vi "Main.vi"(11 "Module Admin":refnum<class "Delacor_lib_QMH_Module Admin.lvclass">) -> ()   [LabVIEW 2020, in "Rename As Application UI.lvlib"]
doc: "This template is based off of the Queued Message Handler design pattern and the Queued Message Handler project template that ships with LabVIEW.\n\nThe main difference is that the queue is private to this module and communication between modules is performed via Broadcast and Request events.\n\nRequest events are wrapped in public API methods and are handled in the Event Handling Loop (EHL) of this VI. Any module can register for Broadcast events sent by this module. The EHL generates messages based on user interface actions.\n\nThe Message Handling Loop (MHL) processes messages generated by the EHL, or by other messages. The messages are string values, so new messages can be added easily to the Message Cases case structure in the MHL. Each message cluster can also provide an optional value for Message Data, which is a variant that can be converted to whatever message-specific data is required.\n_____\nBased on DQMH Project Template 6.1.0.94.\n\n<b>Note:</b> This VI was modified by the <b>Validate DQMH Module</b> tool to add a call to the Error Reported VI at the end of the 'Exit' MHL frame."
uses:
  Rename As Application UI.lvlib
  <vilib>/Delacor/Delacor QMH/Libraries/Module Admin_class/Delacor_lib_QMH_Module Admin.lvclass
  Module Data--cluster.ctl
  Configuration/Configuration--cluster.ctl
  <vilib>/Delacor/Delacor QMH/Libraries/Message Queue_class/Delacor_lib_QMH_Message Queue.lvclass/Delacor_lib_QMH_Message Queue.ctl
  Stop Argument--cluster.ctl
  <vilib>/Utility/miscctls.llb/LVPointTypeDef.ctl
  <vilib>/Delacor/Delacor QMH/Libraries/Module Admin_class/Delacor_lib_QMH_Module Admin.lvclass/Delacor_lib_QMH_Module Admin.ctl
  Configuration/Configuration.lvclass
  Configuration/Configuration.lvclass/Configuration.ctl
  <vilib>/Delacor/Delacor QMH/Libraries/Message Queue_class/Delacor_lib_QMH_Enqueue Message (Single).vi
  <vilib>/Delacor/Delacor QMH/Libraries/Module Admin_class/Delacor_lib_QMH_Get External Launch.vi
  Configuration/Get Configuration.vi
  <vilib>/Utility/error.llb/Error Cluster From Error Code.vi
  <vilib>/ErrorRing/Error Ring.xnode
  <vilib>/Delacor/Delacor QMH/Libraries/Message Queue_class/Delacor_lib_QMH_Message Queue.lvclass
  <vilib>/Peloton/Pelobuttons/Pelobuttons_lib_Pelobuttons.lvlib
  <vilib>/Peloton/Peloton Config/DCFG Framework/Peloton_lib_DCFG Framework.lvlib
  Rename As Application Shared/Rename as Application Shared.lvlib
  <vilib>/Peloton/Peloton Config/DCFG Framework/Configuration_class/Configuration.lvclass
panel:
  out "version":string
  in  "About":bool
  in  "Configuration":bool
  in  "Random Path":path
  out "error out":errorcluster
  in  "Simulate MHL Error":bool
  in  "Simulate EHL Error":bool
  # "This will be the main UI for your application.\nIf you are running as an executable and you want to run in debug mode, drag the exe to the cmd prompt and\nadd the argument -- debug.\nThe project already has a build specification."
  # "When editing this GUI, use Pelobuttons."
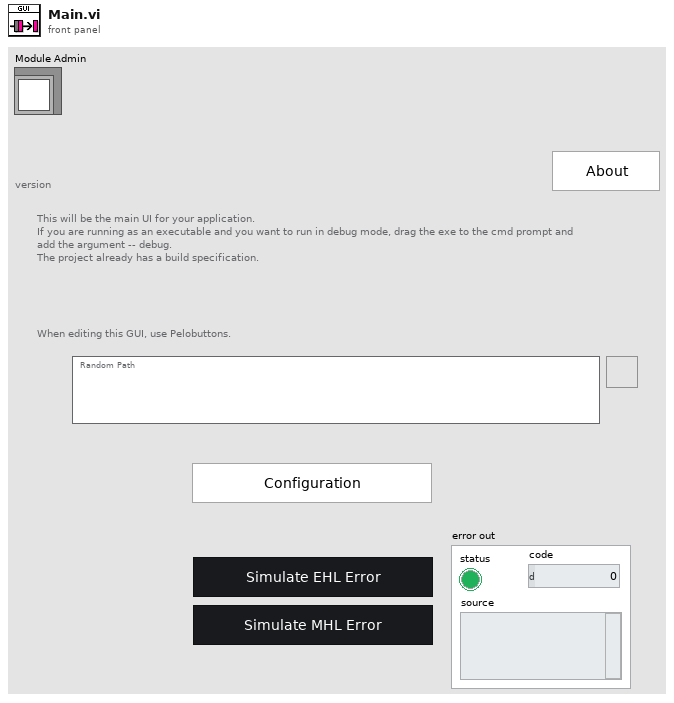
[diagram p1: front panel]
types:
  T1 = typedef "Rename As Application UI.lvlib/Request Events--cluster.ctl" = cluster{"Stop Module":refnum<user-event>, "Show Panel":refnum<user-event>, "Hide Panel":refnum<user-event>, "Get Module Execution Status":refnum<user-event>, "Show Diagram":refnum<user-event>}
  T2 = typedef "Peloton_lib_DCFG Framework.lvlib/Broadcast Events--cluster.ctl" = cluster{"Module Did Init":refnum<user-event>, "Status Updated":refnum<user-event>, "Error Reported":refnum<user-event>, "Module Did Stop":refnum<user-event>, "Update Module Execution Status":refnum<user-event>, "View Changed":refnum<user-event>, "Main Window Closed":refnum<user-event>, "Configuration Committed":refnum<user-event>, "Configuration Canceled":refnum<user-event>, "Views List Updated":refnum<user-event>, "Config Folder Path Updated":refnum<user-event>}
  T3 = typedef "Rename As Application UI.lvlib/Module Data--cluster.ctl" = cluster{"Status":string, "Configuration":T4}
  T4 = typedef "Rename As Application UI.lvlib/Configuration.lvclass/Configuration--cluster.ctl" = cluster{"Random Path":path}
  T5 = enum32{"invalid lock state", "Not Locked", "Locked (No Password)", "Password-protected"}
  T6 = typedef "Rename As Application UI.lvlib/Stop Argument--cluster.ctl" = cluster{"Origin":string, "Exit via Stop Module Req?":bool, "Wait for Module to stop?":bool}
  T7 = typedef "LVPointTypeDef.ctl" = cluster{"Horizontal":i16, "Vertical":i16}
  T8 = enum32{"Invalid", "Standard", "Closed", "Hidden", "Minimized", "Maximized"}
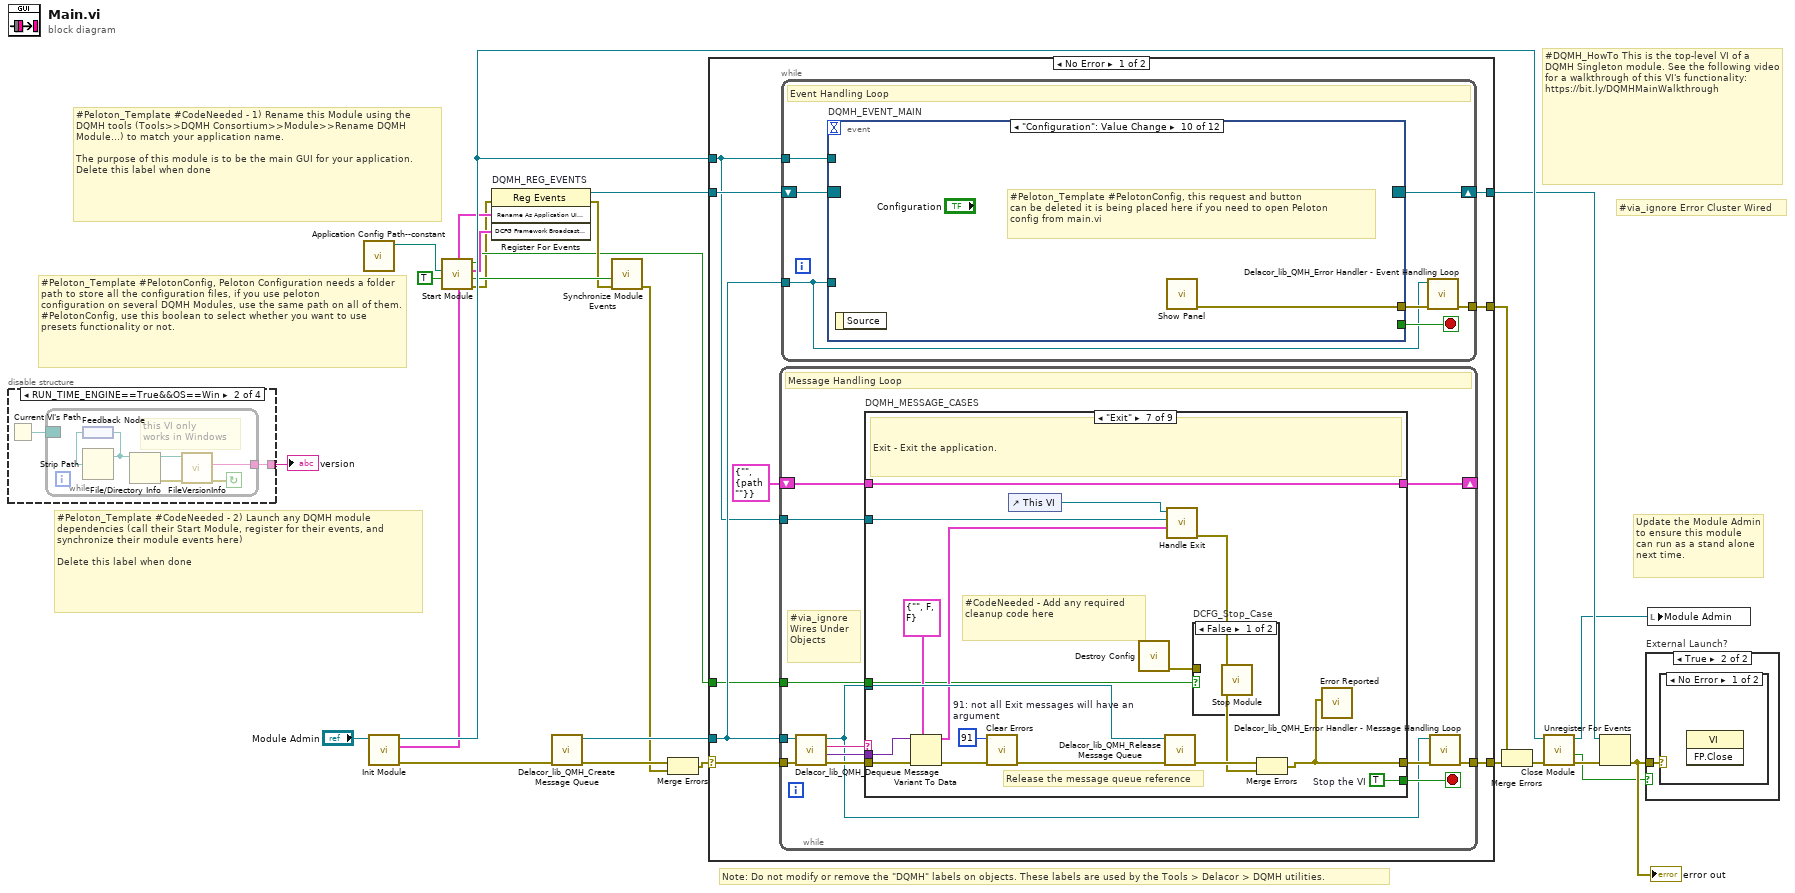
[diagram p0: block diagram]
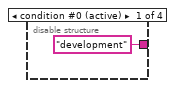
[diagram p2: hidden frame]
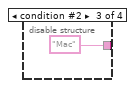
[diagram p3: hidden frame]
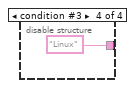
[diagram p4: hidden frame]
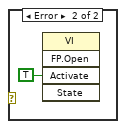
[diagram p6: hidden frame]
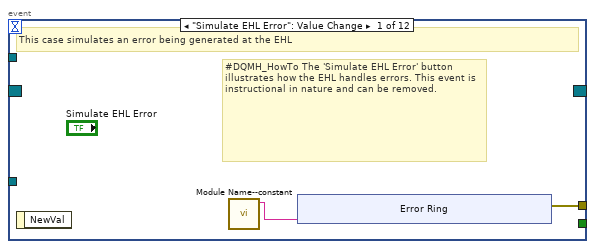
[diagram p7: hidden frame]
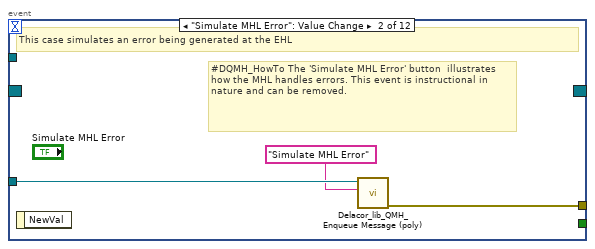
[diagram p8: hidden frame]
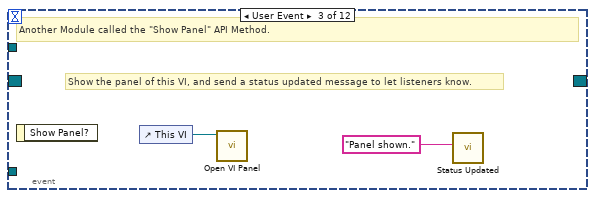
[diagram p9: hidden frame]
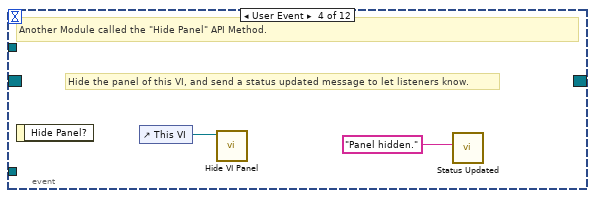
[diagram p10: hidden frame]
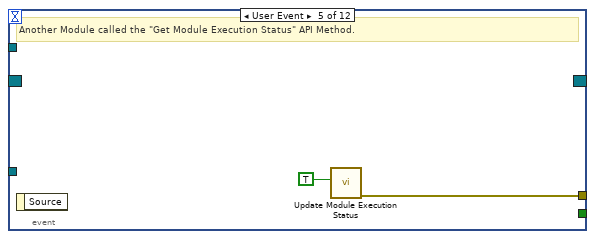
[diagram p11: hidden frame]
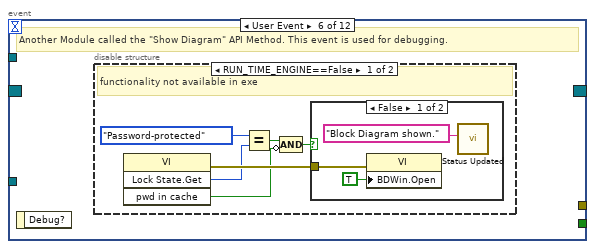
[diagram p12: hidden frame]
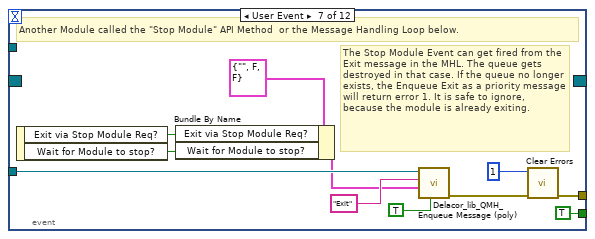
[diagram p15: hidden frame]
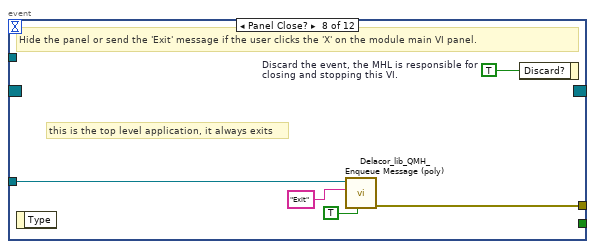
[diagram p16: hidden frame]
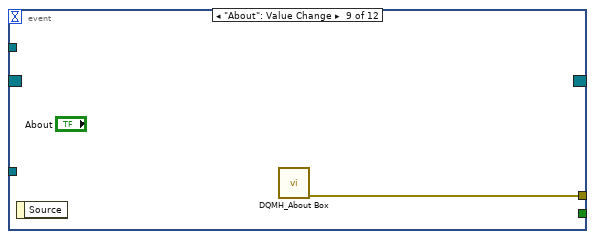
[diagram p17: hidden frame]
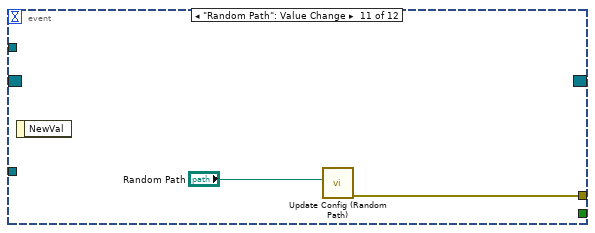
[diagram p18: hidden frame]
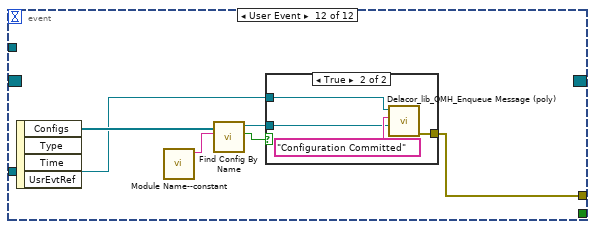
[diagram p19: hidden frame]
diagram:
  # "#Peloton_Template #PelotonConfig, Peloton Configuration needs a folder path to store all the configuration files, if you use peloton\nconfiguration on several DQMH Modules, use the same path on all of them.\n#PelotonConfig, use this boolean to select whether you want to use\npresets functionality or not."
  # "#via_ignore Error Cluster Wired"
  # "#Peloton_Template #CodeNeeded - 2) Launch any DQMH module dependencies (call their Start Module, register for their events, and synchronize their module events here)\n\nDelete this label when done"
  # "#Peloton_Template #CodeNeeded - 1) Rename this Module using the DQMH tools (Tools>>DQMH Consortium>>Module>>Rename DQMH Module...) to match your application name.\n\nThe purpose of this module is to be the main GUI for your application.\nDelete this label when done"
  # "#DQMH_HowTo This is the top-level VI of a DQMH Singleton module. See the following video for a walkthrough of this VI's functionality: https://bit.ly/DQMHMainWalkthrough"
  # "Note: Do not modify or remove the \"DQMH\" labels on objects. These labels are used by the Tools > Delacor > DQMH utilities."
  # "Update the Module Admin to ensure this module can run as a stand alone next time."
  n1 = disable-structure "Conditional Disable Structure" shown="RUN_TIME_ENGINE==True&&OS==Win" {
    disable-tunnel: ["development" w27 "Mac" "Linux"] -> w9
    frame condition #0 (active) {
    }
    frame condition #1 {
      n2 = Current VI's Path() -> (path=w28:path)
      n3 = while {
        border: w28 -> [_]
        tunnel: [w29] -> w27
        stop <- w33 continue-if-true
        # "this VI only \nworks in Windows"
        n4 = feedback #1() -> (w32:path)
        n5 = Strip Path(path=w32) -> (stripped path=w31:path)  [unwired: 1 out]
        n6 = feedback-in #1(w31) -> ()
        n7 = File/Directory Info(path=w31) -> (path out=w30:path, error out=w34:errorcluster)  [unwired: 1 in, 5 out]
        n8 = call <vilib>:"FileVersionInfo.vi"("error in (no error)"=w34, "Application Path in"=w30) -> ("error out"=w33:errorcluster, "File Version Info"=w29:string)  [unwired: 6 in, 2 out]
      }
    }
    frame condition #2 {
    }
    frame condition #3 {
    }
  }
  "version" <- w9
  n9 = call "Application Config Path--constant.vi"() -> ("File Path"=w2:path)  [unwired: 11 in]
  n10 = call "Init Module.vi"("Singleton Module Admin in"="Module Admin") -> ("error out"=w24:errorcluster, "Rename As Application UI Request Events"=w14:T1, "Singleton Module Admin out"=w17:refnum<class "Delacor_lib_QMH_Module Admin.lvclass">)  [unwired: 8 in]
  n11 = call <vilib>:"Start Module.vi"("Enable Presets (F)"=TRUE, "Config Folder"=w2) -> ("error out"=w1:errorcluster, "Wait for Event Sync?"=w7:bool, "DCFG Framework Broadcast Events"=w8:T2, "Module Was Already Running?"=w4:bool)  [unwired: 6 in]
  n12 = register-events "DQMH_REG_EVENTS"(error in=w1, w14, w8) -> (reference out=w15:refnum<event-registration>, error out=w6:errorcluster)  [unwired: 1 in]
  n13 = call <vilib>:"Delacor_lib_QMH_Create Message Queue.vi"("error in"=w24) -> ("error out"=w19:errorcluster, "Message Queue"=w13:refnum<class "Delacor_lib_QMH_Message Queue.lvclass">)  [unwired: 9 in]
  n14 = call <vilib>:"Synchronize Module Events.vi"("error in (no error)"=w6, "Wait for Event Sync?"=w7) -> ("error out"=w5:errorcluster)  [unwired: 9 in]
  n15 = Merge Errors(w19, w5) -> (w18:errorcluster)
  n16 = case shown="No Error" w18 {
    selector: w18 -> [w43 w229]
    tunnel: [w45 w228] -> w25
    tunnel: [w42 w227] -> w16
    tunnel: w15 -> [w40 w227]
    tunnel: w13 -> [w39 w222]
    tunnel: [w44 _] -> w22
    tunnel: w17 -> [w38 w223]
    tunnel: w4 -> [w37 w221]
    frame No Error {
      n17 = while {
        tunnel: w39 -> [w113]
        shift-right: [w117] -> _
        shift-left: T3 {"Status"="", "Configuration"={"Random Path"=path ""}} ("Data Cluster") -> [w118]
        tunnel: w43 -> [w121]
        tunnel: [w119] -> w45
        tunnel: w38 -> [w111]
        tunnel: w37 -> [w110]
        stop <- w116 stop-if-true
        # "#via_ignore Wires Under Objects"
        # "Message Handling Loop"
        n18 = call-dynamic "Delacor_lib_QMH_Dequeue Message.vi"("error in"=w121, "Message Queue in"=w113) -> ("error out"=w120:errorcluster, "Message Data"=w114:variant, "Message"=w115:string, "Message Queue out"=w112:refnum<class "Delacor_lib_QMH_Message Queue.lvclass">)  [unwired: 6 in]
        n19 = case "DQMH_MESSAGE_CASES" shown="\"Exit\"" w115 {
          selector: w115 -> [_ _ _ _ _ _ _ w199 _]
          tunnel: w112 -> [_ _ _ _ _ w167 w190 _ _]
          tunnel: w120 -> [w143 w147 w150 w152 w157 w174 w197 w201 w220]
          tunnel: [w142 w147 w149 w152 w156 w170 w194 w202 w217] -> w122
          tunnel: w118 -> [w129 w146 w148 w151 w154 w169 w189 w200 w219]
          tunnel: [w128 w146 w148 w151 w154 w169 w189 w200 w218] -> w117
          tunnel: [_ _ _ _ _ _ w188 _ _] -> w116
          tunnel: w114 -> [_ _ _ _ _ w168 w191 _ w216]
          tunnel: w111 -> [w134 _ _ _ _ w166 w184 _ _]
          tunnel: w110 -> [_ _ _ _ _ _ w181 _ _]
          frame "Initialize" {
            # "#CodeNeeded - Initialize the appearance of the front panel."
            # "Initialize - Any operation that needs to be done before the module can receive messages. Synchronize Caller Events.vi will inform Start Module.vi that the module has launched and is ready to receive messages. Module Did Init.vi will broadcast that the module initialized."
            n20 = call "Synchronize Caller Events.vi"("error in (no error)"=w143, "Singleton Module Admin in"=w134) -> ("error out"=w125:errorcluster, "Singleton Module Admin out"=w131:refnum<class "Delacor_lib_QMH_Module Admin.lvclass">)  [unwired: 8 in]
            n21 = property on="Property Node" class="Module Admin"(reference=w131) -> ("Accessors:External Launch"=w138:bool)  [unwired: 1 in, 2 out]
            n22 = flat-sequence {
              tunnel: w125 -> [_]
              frame #0 {
                n23 = call <vilib>:"Brand UI - FP.vi"() -> ()  [unwired: 12 in]
              }
            }
            n24 = call "Init Config.vi"("error in"=w125) -> ("error out"=w126:errorcluster, "Configuration"=w124:T4)  [unwired: 9 in]
            n25 = Select(t=T8."Hidden" ("State"), s=w138, f=T8."Standard" ("State")) -> (s? t:f=w135:T8)
            n26 = call "Module Name--constant.vi"() -> ("Module Name"=w141:string)  [unwired: 11 in]
            n27 = Unbundle By Name(w124) -> ("Random Path"=w123:path)
            n28 = property on="Property Node" class="VI"("Front Panel.Title"=w141) -> (reference out=w140:refnum<vi>, error out=w145:errorcluster)  [unwired: 2 in]
            n29 = call "Module Name--constant.vi"() -> ("Module Name"=w132:string)  [unwired: 11 in]
            n30 = invoke on="Invoke Node" class="VI" method="FP.Open"(reference=w140, error in=w145, "State"=w135) -> (reference out=w139:refnum<vi>, error out=w144:errorcluster)  [unwired: 2 in, 3 out]
            n31 = Bundle By Name(cluster=w129, "Status"="Init", "Configuration"=w124) -> (w128:T3)
            n32 = local write "Random Path"(w123) -> ()
            n33 = call "Module Did Init.vi"("error in (no error)"=w126, "Initialized?"=TRUE, "Origin"=w132) -> ("error out"=w142:errorcluster)  [unwired: 8 in]
            n34 = invoke on="Invoke Node" class="VI" method="FP.Center"(reference=w139, error in=w144) -> ()  [unwired: 1 in, 3 out]
            n35 = property on="Pane" class="Pane"("Origin"=T7 {"Horizontal"=0, "Vertical"=0}) -> ()  [unwired: 2 in, 2 out]
          }
          frame "---Module Specific---" {
            # "Separator -- The following cases handle messages specific to this Module."
          }
          frame "---Copy This Frame---" {
            # "Duplicate this frame when creating new messages.  Change this comment in the duplicated frame to describe this message."
            n36 = Merge Errors(w150) -> (w149:errorcluster)
          }
          frame "---Exit and Error Handling---" {
            # "Separator - The following cases handle errors and exit messages."
          }
          frame "Simulate MHL Error" {
            # "#DQMH_HowTo The 'Simulate MHL Error' button  illustrates how the MHL handles errors. This event is instructional in nature and can be removed."
            # "Simulate an error occurring at the MHL"
            n37 = call "Module Name--constant.vi"() -> ("Module Name"=w153:string)  [unwired: 11 in]
            n38 = xnode ("Error Ring")("parameter 0"=w153) -> ("error out"=w155:errorcluster)
            n39 = Merge Errors(w157, w155) -> (w156:errorcluster)
          }
          frame "Error" {
            # "#CodeRecommended - If you ever change the name of this \"Error\" message, you'll need to update the name in the Check Loop Error.vi as well."
            # "#CodeRecommended - If the module is running in standalone mode (External Launch = FALSE), this code will pop up an error dialog and call the 'Exit' message if an error occurs. Add more fine-grained error handling here."
            # "Error - Check the error message data and respond accordingly. This message is sent by the \"Error Handler\" VIs at the end of each loop in this application."
            n40 = property on="Property Node" class="Module Admin"(reference=w166) -> ("Accessors:External Launch"=w165:bool)  [unwired: 1 in, 2 out]
            n41 = Variant To Data(error in=w174, type=errorcluster {"status"=FALSE, "code"=0, "source"=""} ("error constant"), Variant=w168) -> (data=w175:errorcluster, error out=w172:errorcluster)
            n42 = call "Error Reported.vi"("Error"=w175) -> ()  [unwired: 10 in, 1 out]
            n43 = case shown="False" w165 {
              tunnel: [w180 _] -> w171
              tunnel: w167 -> [w178 _]
              tunnel: w175 -> [w179 _]
              frame False {
                # "If the module is running standalone, then pop up an error dialog and call the \"Exit\" message."
                n44 = call <vilib>:"Simple Error Handler.vi"("error in (no error)"=w179) -> ()  [unwired: 4 in, 5 out]
                n45 = call-poly <vilib>:"Delacor_lib_QMH_Enqueue Message (poly).vi"("Priority Message? (F)"=TRUE, "Message"="Exit", "Message Queue in"=w178) -> ("error out"=w180:errorcluster)  [unwired: 7 in, 1 out]
              }
              frame True {
                # "If the module was launched externally, calling the Error Reported broadcast VI is the only action performed by the \"Error\" message. The module's caller can then process the error appropriately."
              }
            }
            n46 = Merge Errors(w172, w171) -> (w170:errorcluster)
            n47 = local write "error out"(w170) -> ()
          }
          frame "Exit" {
            w187 = 91  # 91: not all Exit messages will have an argument
            w188 = TRUE  # Stop the VI
            # "Release the message queue reference"
            # "#CodeNeeded - Add any required cleanup code here"
            # "Exit - Exit the application."
            n48 = Variant To Data(error in=w197, type=T6 {"Origin"="", "Exit via Stop Module Req?"=FALSE, "Wait for Module to stop?"=FALSE} ("Stop Argument"), Variant=w191) -> (data=w185:T6, error out=w193:errorcluster)
            n49 = call <vilib>:"Clear Errors.vi"("error in (no error)"=w193, "specific error code to clear (0: all)"=w187) -> ("error out"=w196:errorcluster)  [unwired: 4 in, 1 out]
            n50 = control-ref of="This VI"() -> (w183:refnum<vi>)
            n51 = call "Destroy Config.vi"() -> ("error out"=w182:errorcluster)  [unwired: 11 in]
            n52 = call-dynamic "Delacor_lib_QMH_Release Message Queue.vi"("error in"=w196, "Message Queue"=w190) -> ("error out"=w195:errorcluster)  [unwired: 9 in]
            n53 = call "Handle Exit.vi"("Stop Argument"=w185, "Admin in"=w184, "VI reference"=w183) -> ("error out"=w192:errorcluster)  [unwired: 7 in, 1 out]
            n54 = case "DCFG_Stop_Case" shown="False" w181 {
              tunnel: w182 -> [_ _]
              frame False {
                n55 = call <vilib>:"Stop Module.vi"() -> ()  [unwired: 11 in, 1 out]
              }
              frame True {
                # "Let DCFG Running if it was already running"
              }
            }
            n56 = Merge Errors(w195, w192) -> (w194:errorcluster)
            n57 = call "Error Reported.vi"("Error"=w194) -> ()  [unwired: 10 in, 1 out]
          }
          frame Default {
            # "'Default' case only runs if there is a message that isn't defined in any of the other cases.  Output a programming error."
            n58 = call "Module Name--constant.vi"() -> ("Module Name"=w198:string)  [unwired: 11 in]
            n59 = xnode ("Error Ring")("parameter 0"=w199, "parameter 1"=w198) -> ("error out"=w203:errorcluster)
            n60 = Merge Errors(w201, w203) -> (w202:errorcluster)
          }
          frame "Configuration Committed" {
            w215 = refnum<class "Configuration.lvclass"> refnum  # Module_Config_Class
            n61 = Variant To Data(error in=w220, type=w215, Variant=w216) -> (data=w214:refnum<class "Configuration.lvclass">, error out=w217:errorcluster)
            n62 = property on="Property Node" class="Config"(reference=w214) -> ("Accessors:Configuration"=w212:T4)  [unwired: 1 in, 2 out]
            n63 = Bundle By Name(cluster=w219, "Configuration"=w212) -> (w218:T3)
            n64 = Unbundle By Name(w212) -> ("Random Path"=w213:path)
            n65 = local write "Random Path"(w213) -> ()
          }
        }
        n66 = call-dynamic "Delacor_lib_QMH_Error Handler - Message Handling Loop.vi"("error in"=w122, "Message Queue in"=w112) -> ("dup error in"=w119:errorcluster)  [unwired: 8 in, 1 out]
      }
      n67 = while {
        tunnel: w39 -> [w46]
        shift-right: [w49] -> w42
        shift-left: w40 -> [w50]
        tunnel: [w51] -> w44
        tunnel: w38 -> [w47]
        stop <- w48 stop-if-true
        # "Event Handling Loop"
        n68 = event "DQMH_EVENT_MAIN" shown="[9] \"Configuration\": Value Change" {
          selector: w50 -> [_ _ _ _ _ _ _ _ _ _ _ _]
          dyn-events: [_ _ _ _ _ _ _ _ _ _ _ _] -> w49
          timeout: _ -> [_ _ _ _ _ _ _ _ _ _ _ _]
          tunnel: [_ _ _ _ _ _ TRUE ("Discard?") _ _ _ _ _] -> w48
          tunnel: w46 -> [_ w63 _ _ _ _ w86 w93 _ _ _ w103]
          tunnel: [w54 w64 _ _ w70 _ w89 w95 w96 w97 w98 w105] -> w52
          tunnel: w47 -> [_ _ _ _ _ _ _ _ _ _ _ _]
          event "Simulate EHL Error": Value Change {
            # "#DQMH_HowTo The 'Simulate EHL Error' button  illustrates how the EHL handles errors. This event is instructional in nature and can be removed."
            # "This case simulates an error being generated at the EHL"
            n69 = event-data() -> ()  [unwired: 1 in, 1 out]
            n70 = call "Module Name--constant.vi"() -> ("Module Name"=w53:string)  [unwired: 11 in]
            n71 = xnode ("Error Ring")("parameter 0"=w53) -> ("error out"=w54:errorcluster)
          }
          event "Simulate MHL Error": Value Change {
            # "#DQMH_HowTo The 'Simulate MHL Error' button  illustrates how the MHL handles errors. This event is instructional in nature and can be removed."
            # "This case simulates an error being generated at the EHL"
            n72 = event-data() -> ()  [unwired: 1 in, 1 out]
            n73 = call-poly <vilib>:"Delacor_lib_QMH_Enqueue Message (poly).vi"("Message"="Simulate MHL Error", "Message Queue in"=w63) -> ("error out"=w64:errorcluster)  [unwired: 8 in, 1 out]
          }
          event User Event {
            # "Show the panel of this VI, and send a status updated message to let listeners know."
            # "Another Module called the \"Show Panel\" API Method."
            n74 = event-data() -> ()  [unwired: 1 in, 1 out]
            n75 = control-ref of="This VI"() -> (w66:refnum<vi>)
            n76 = call "Open VI Panel.vi"("VI"=w66) -> ()  [unwired: 10 in, 1 out]
            n77 = call "Status Updated.vi"("Status"="Panel shown." ("format string")) -> ()  [unwired: 10 in, 1 out]
          }
          event User Event {
            # "Hide the panel of this VI, and send a status updated message to let listeners know."
            # "Another Module called the \"Hide Panel\" API Method."
            n78 = event-data() -> ()  [unwired: 1 in, 1 out]
            n79 = control-ref of="This VI"() -> (w68:refnum<vi>)
            n80 = call "Hide VI Panel.vi"("VI"=w68) -> ()  [unwired: 10 in, 1 out]
            n81 = call "Status Updated.vi"("Status"="Panel hidden." ("format string")) -> ()  [unwired: 10 in, 1 out]
          }
          event User Event {
            # "Another Module called the \"Get Module Execution Status\" API Method."
            n82 = event-data() -> ()  [unwired: 1 in, 1 out]
            n83 = call "Update Module Execution Status.vi"("Running?"=TRUE) -> ("error out"=w70:errorcluster)  [unwired: 10 in]
          }
          event User Event {
            # "Another Module called the \"Show Diagram\" API Method. This event is used for debugging."
            n84 = event-data() -> ()  [unwired: 1 in, 1 out]
            n85 = disable-structure shown="RUN_TIME_ENGINE==False" {
              frame condition #0 (active) {
                # "functionality not available in exe"
                n86 = invoke on="Invoke Node" class="VI" method="Lock State.Get"() -> (error out=w76:errorcluster, "Get Lock State"=w75:T5, "pwd in cache"=w72:bool)  [unwired: 4 in, 1 out]
                n87 = Equal?(x=T5."Password-protected", y=w75) -> (x = y?=w73:bool)
                n88 = Compound Arithmetic op=AND(w73, invert w72) -> (w71:bool)
                n89 = case shown="False" w71 {
                  tunnel: w76 -> [w79 _]
                  frame False {
                    n90 = property on="Property Node" class="VI"(error in=w79, "BDWin.Open"=TRUE ("Block Diagram Window:Open")) -> ()  [unwired: 1 in, 2 out]
                    n91 = call "Status Updated.vi"("Status"="Block Diagram shown." ("format string")) -> ()  [unwired: 10 in, 1 out]
                  }
                  frame True {
                    # "Password-protected VI, and the password is not in the cache. Do not show the diagram."
                  }
                }
              }
              frame condition #1 {
              }
            }
          }
          event User Event {
            # "The Stop Module Event can get fired from the Exit message in the MHL. The queue gets destroyed in that case. If the queue no longer exists, the Enqueue Exit as a priority message will return error 1. It is safe to ignore, because the module is already exiting."
            # "Another Module called the \"Stop Module\" API Method  or the Message Handling Loop below."
            n92 = event-data() -> ("Exit via Stop Module Req?"=w82:bool, "Wait for Module to stop?"=w81:bool)  [unwired: 1 in]
            n93 = Bundle By Name(cluster=T6 {"Origin"="", "Exit via Stop Module Req?"=FALSE, "Wait for Module to stop?"=FALSE} ("Stop Argument"), "Exit via Stop Module Req?"=w82, "Wait for Module to stop?"=w81) -> (w80:T6)
            n94 = call-poly <vilib>:"Delacor_lib_QMH_Enqueue Message (poly).vi"("Priority Message? (F)"=TRUE, "Message Data"=w80, "Message"="Exit", "Message Queue in"=w86) -> ("error out"=w90:errorcluster)  [unwired: 6 in, 1 out]
            n95 = call <vilib>:"Clear Errors.vi"("error in (no error)"=w90, "specific error code to clear (0: all)"=1) -> ("error out"=w89:errorcluster)  [unwired: 4 in, 1 out]
          }
          event Panel Close? {
            w94 = TRUE  # Discard the event, the MHL is responsible for closing and stopping this VI.
            # "this is the top level application, it always exits"
            # "Hide the panel or send the 'Exit' message if the user clicks the 'X' on the module main VI panel."
            n96 = event-data() -> ()  [unwired: 1 in, 1 out]
            n97 = call-poly <vilib>:"Delacor_lib_QMH_Enqueue Message (poly).vi"("Priority Message? (F)"=TRUE, "Message"="Exit", "Message Queue in"=w93) -> ("error out"=w95:errorcluster)  [unwired: 7 in, 1 out]
            n98 = event-data ("Event Filter Node")("Discard?"=w94) -> ()  [unwired: 1 in, 1 out]
          }
          event "About": Value Change {
            n99 = event-data() -> ()  [unwired: 1 in, 1 out]
            n100 = call <vilib>:"DQMH_About Box.vi"() -> ("error out"=w96:errorcluster)  [unwired: 11 in]
          }
          event "Configuration": Value Change {
            # "#Peloton_Template #PelotonConfig, this request and button\ncan be deleted it is being placed here if you need to open Peloton\nconfig from main.vi"
            n101 = event-data() -> ()  [unwired: 1 in, 1 out]
            n102 = call <vilib>:"Show Panel.vi"() -> ("error out"=w97:errorcluster)  [unwired: 11 in]
          }
          event "Random Path": Value Change {
            n103 = event-data() -> ()  [unwired: 1 in, 1 out]
            n104 = call "Update Config (Random Path).vi"("Random Path"="Random Path") -> ("error out"=w98:errorcluster)  [unwired: 10 in]
          }
          event User Event {
            n105 = event-data() -> ("Configs"=w104:refnum<class "Configuration.lvclass">[])  [unwired: 1 in, 3 out]
            n106 = call "Module Name--constant.vi"() -> ("Module Name"=w102:string)  [unwired: 11 in]
            n107 = call <vilib>:"Find Config By Name.vi"("Config Name"=w102, "All Config Classes"=w104) -> ("Found"=w101:bool, "Configuration"=w100:refnum<class "Configuration.lvclass">)  [unwired: 6 in, 2 out]
            n108 = case shown="True" w101 {
              tunnel: w103 -> [_ w108]
              tunnel: [_ w109] -> w105
              tunnel: w100 -> [_ w106]
              frame False {
              }
              frame True {
                n109 = call-poly <vilib>:"Delacor_lib_QMH_Enqueue Message (poly).vi"("Message Data"=w106, "Message"="Configuration Committed", "Message Queue in"=w108) -> ("error out"=w109:errorcluster)  [unwired: 7 in, 1 out]
              }
            }
          }
        }
        n110 = call-dynamic "Delacor_lib_QMH_Error Handler - Event Handling Loop.vi"("error in"=w52, "Message Queue in"=w46) -> ("dup error in"=w51:errorcluster)  [unwired: 8 in, 1 out]
      }
    }
    frame Error {
      # "Synchronize Caller Events.vi will inform Start Module.vi that the module has launched and will let the code calling Start Module.vi register for broadcasts and would permit the caller receive the broadcast that an error occurred at launch time."
      n111 = call-dynamic "Delacor_lib_QMH_Release Message Queue.vi"("error in"=w229, "Message Queue"=w222) -> ("error out"=w228:errorcluster)  [unwired: 9 in]
      n112 = call "Synchronize Caller Events.vi"("Singleton Module Admin in"=w223) -> ("error out"=w230:errorcluster)  [unwired: 9 in, 1 out]
      n113 = call "Module Name--constant.vi"() -> ("Module Name"=w226:string)  [unwired: 11 in]
      n114 = Format Into String(format string="An error occurred during initialization. %s is no longer running.", w226) -> (resulting string=w224:string)  [unwired: 2 in, 1 out]
      n115 = Merge Errors(w228, w230) -> (w231:errorcluster)
      n116 = case "DCFG_Stop_Case" shown="False" w221 {
        frame False {
          n117 = call <vilib>:"Stop Module.vi"() -> ()  [unwired: 11 in, 1 out]
        }
        frame True {
          # "Let DCFG Running if it was already running"
        }
      }
      n118 = call "Error Reported.vi"("Additional Information"=w224, "Error"=w231) -> ()  [unwired: 9 in, 1 out]
    }
  }
  n119 = Merge Errors(w22, w25) -> (w21:errorcluster)
  n120 = call "Close Module.vi"("error in (no error)"=w21, "Module Admin in"=w17) -> ("error out"=w23:errorcluster, "External Launch"=w10:bool, "Module Admin out"=w11:refnum<class "Delacor_lib_QMH_Module Admin.lvclass">)  [unwired: 7 in]
  n121 = Unregister For Events(event registration refnum=w16, error in=w23) -> (error out=w20:errorcluster)
  "error out" <- w20
  n122 = case "External Launch?" shown="True" w10 {
    tunnel: w20 -> [_ w232]
    frame False {
    }
    frame True {
      n123 = case shown="No Error" w232 {
        frame No Error {
          n124 = invoke on="Invoke Node" class="VI" method="FP.Close"() -> ()  [unwired: 3 in, 3 out]
        }
        frame Error {
          n125 = invoke on="Invoke Node" class="VI" method="FP.Open"("Activate"=TRUE ("Activate?")) -> ()  [unwired: 4 in, 5 out]
        }
      }
    }
  }
  n126 = local write "Module Admin"(w11) -> ()
